vi "Telescope Configure GUI.vi"(8 "error in (no error)":errorcluster, 10 "Telescope Name":string="Default", 11 "LDT Telescope in":refnum<class "LDT Telescope.lvclass">) -> (0 "error out":errorcluster, 3 "LDT Telescope out":refnum<class "LDT Telescope.lvclass">)   [LabVIEW 2022 SP3, in "LDT Telescope.lvclass"]
uses:
  LDT Telescope.lvclass
  LDT Telescope.lvclass/LDT Telescope.ctl
  Telescope.lvclass
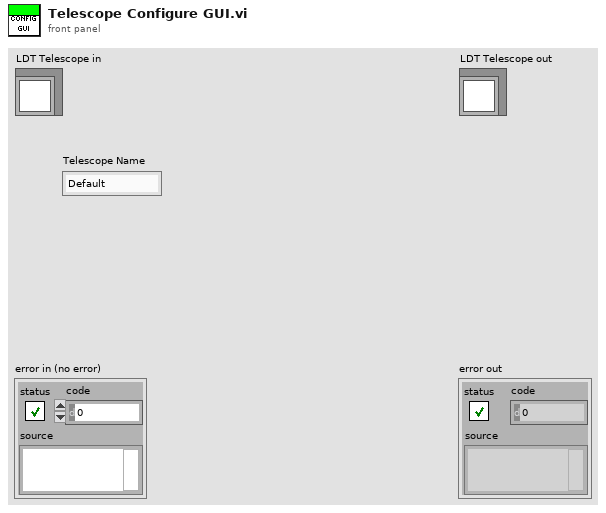
[diagram p1: front panel]
types:
  T1 = typedef "LDT Telescope.lvclass/typedef cluster LDT Telescope Settings.ctl" = cluster{"host":string, "port":string}
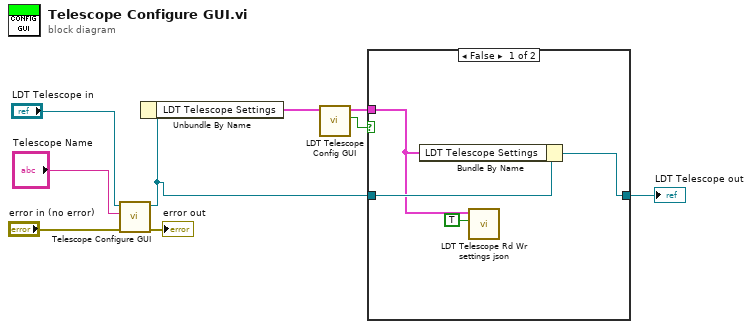
[diagram p0: block diagram]
diagram:
  n1 = call-parent "Telescope Configure GUI.vi"("error in (no error)"="error in (no error)", "Telescope Name"="Telescope Name", "Telescope in"="LDT Telescope in") -> ("error out"=→"error out":errorcluster, "Telescope out"=w3:refnum<class "LDT Telescope.lvclass">)  [unwired: 7 in]
  n2 = Unbundle By Name(w3) -> ("LDT Telescope Settings"=w5:T1)
  n3 = call "LDT Telescope Config GUI.vi"("LDT Telescope Settings"=w5) -> ("cancelled"=w4:bool, "LDT Telescope Settings out"=w1:T1)  [unwired: 9 in]
  n4 = case shown="False" w4 {
    tunnel: w3 -> [w13 w14]
    tunnel: [w12 w14] -> w2
    tunnel: w1 -> [w11 _]
    frame False {
      n5 = Bundle By Name(cluster=w13, "LDT Telescope Settings"=w11) -> (w12:refnum<class "LDT Telescope.lvclass">)
      n6 = call "LDT Telescope Rd Wr settings json.vi"("Write? (F:Read)"=TRUE, "LDT Telescope Settings"=w11) -> ()  [unwired: 8 in, 2 out]
    }
    frame True {
    }
  }
  "LDT Telescope out" <- w2
